vi "Comman1_Main(RemoteLoader).vi"() -> ()   [LabVIEW 2020]
uses:
  RemoteControl_class/RemoteControl.lvclass
  Light_class/Light.lvclass
  GarageDoor_class/GarageDoor.lvclass
  CeilingFan_class/CeilingFan.lvclass
  LightOnCommand_class/LightOnCommand.lvclass
  C:/Projects/OpenGDS_DesignPatterns/Command1/Command_class/Command.lvclass
  LightOffCommand_class/LightOffCommand.lvclass
  GarageDoorOpenCommand_class/GarageDoorOpenCommand.lvclass
  GarageDoorCloseCommand_class/GarageDoorCloseCommand.lvclass
  CeilingFanHighCommand_class/CeilingFanHighCommand.lvclass
  CeilingFanLowCommand_class/CeilingFanLowCommand.lvclass
  Command_class/Command.lvclass
panel:
  in  "stop":bool
  out "error out":errorcluster
  in  "error in (no error)":errorcluster
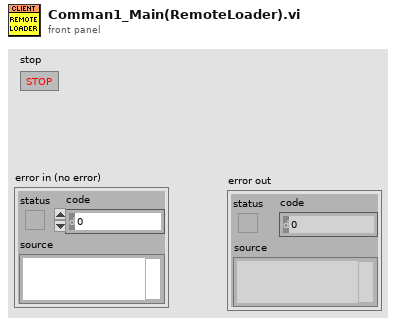
[diagram p1: front panel]
types:
  T1 = cluster{"Remote":refnum<class "RemoteControl.lvclass">, "Light":refnum<class "Light.lvclass">, "GarageDoor":refnum<class "GarageDoor.lvclass">, "CeilingFan":refnum<class "CeilingFan.lvclass">}
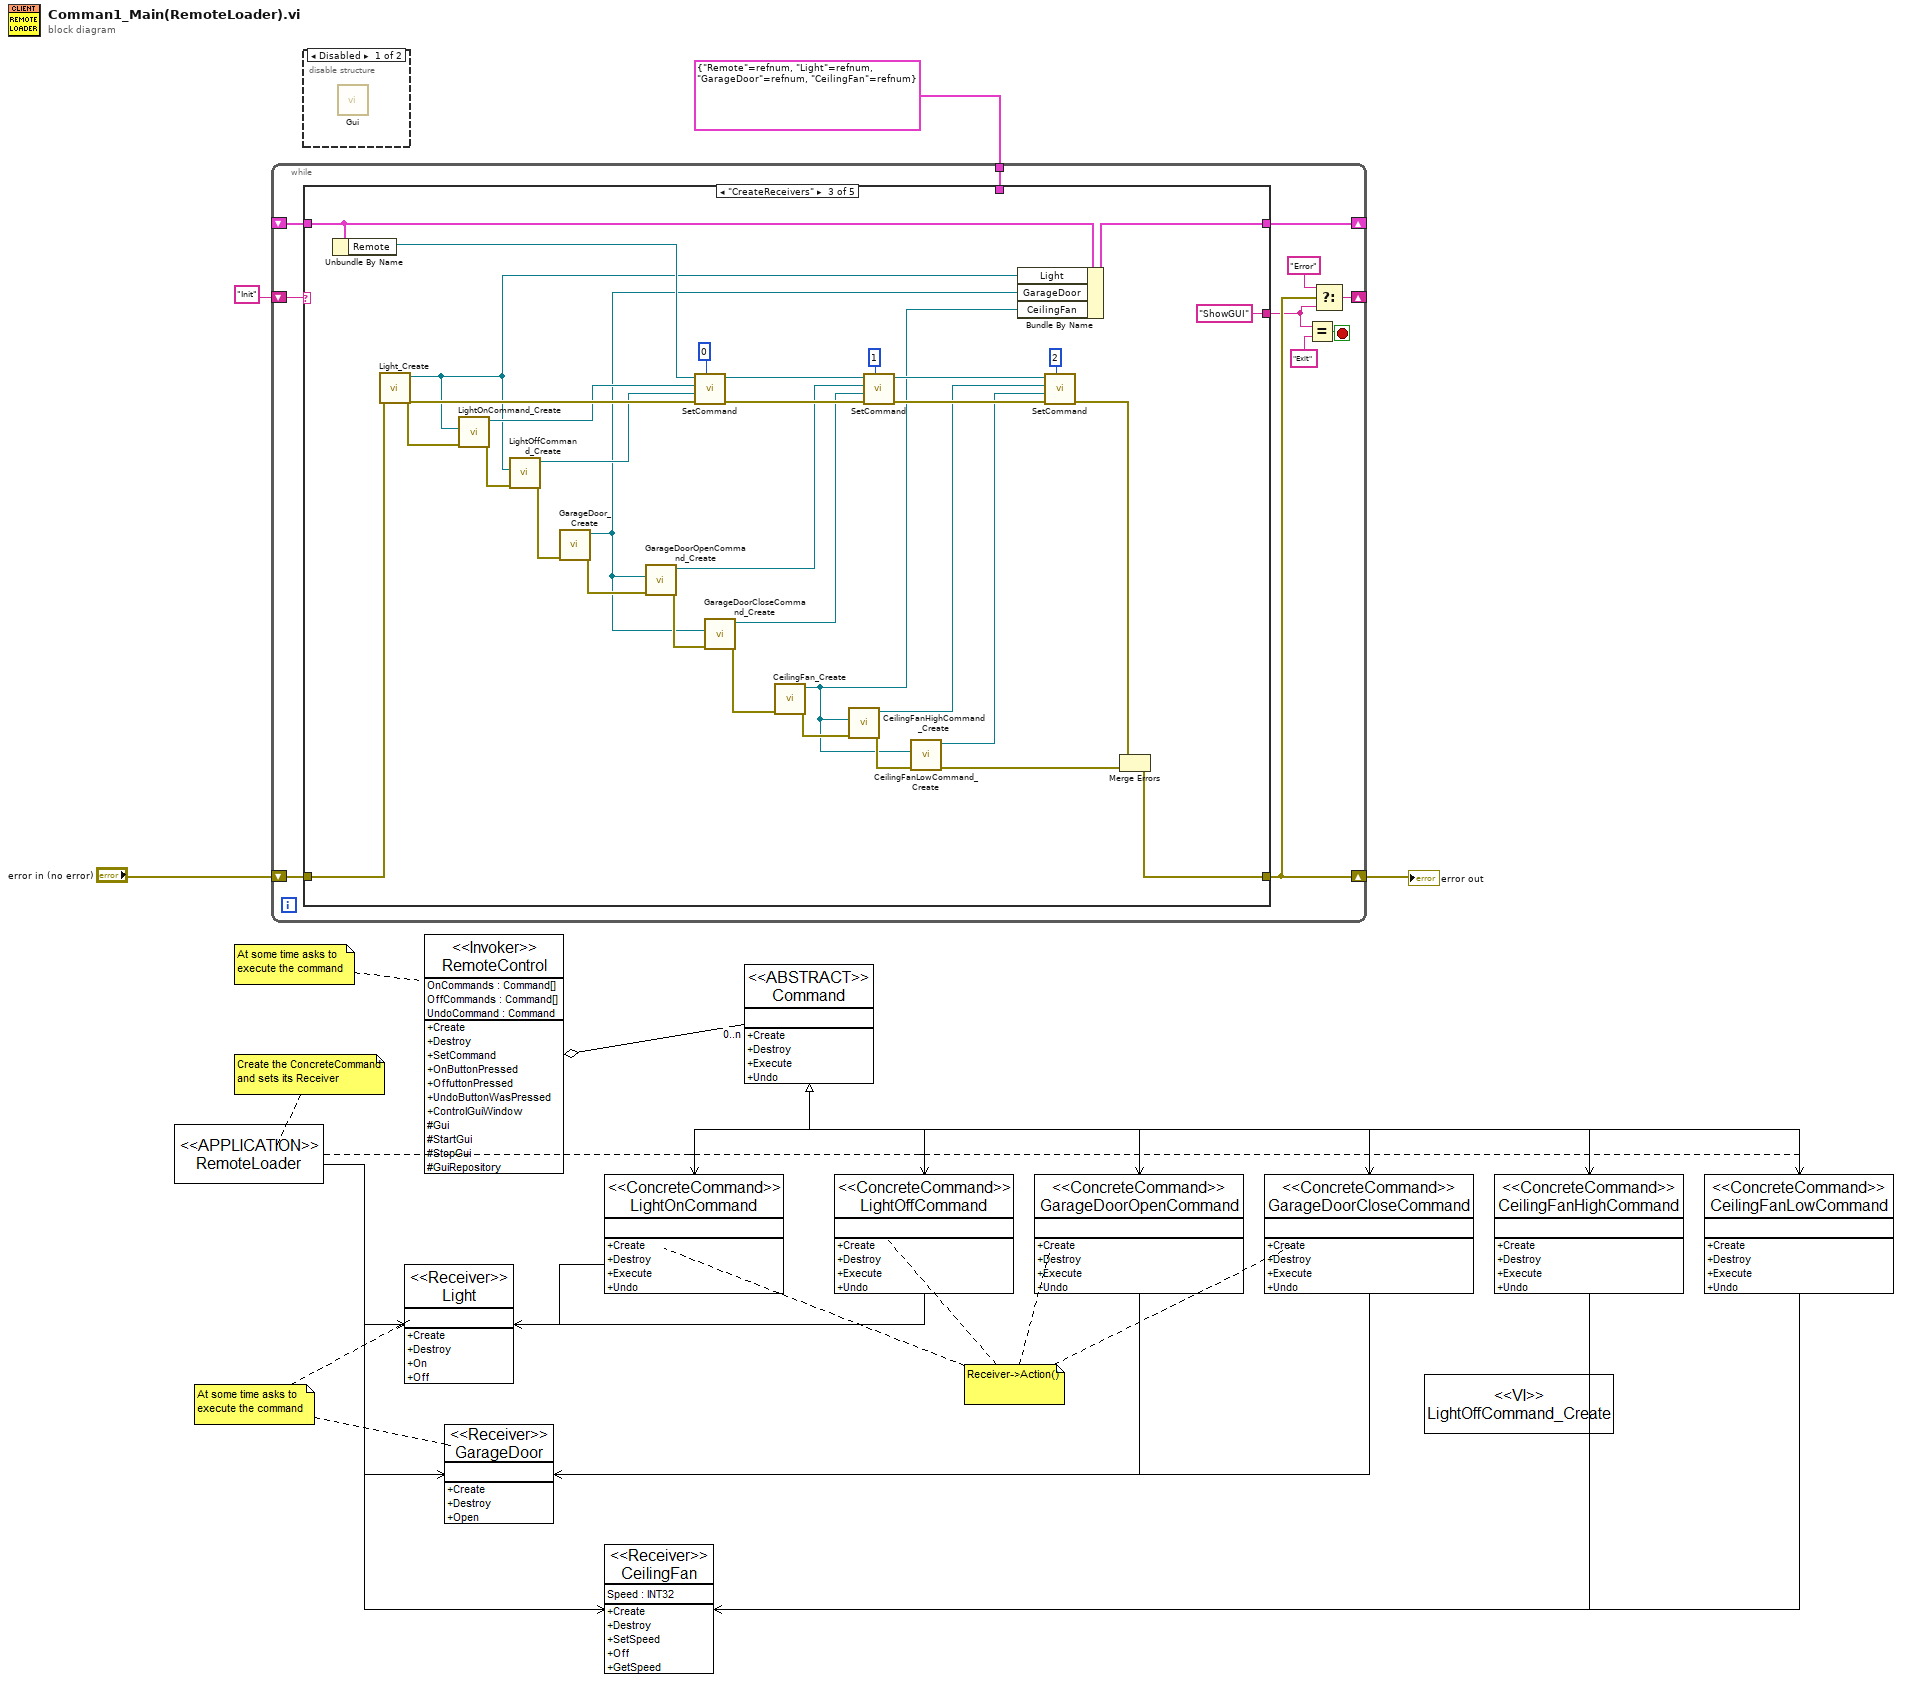
[diagram p0: block diagram]
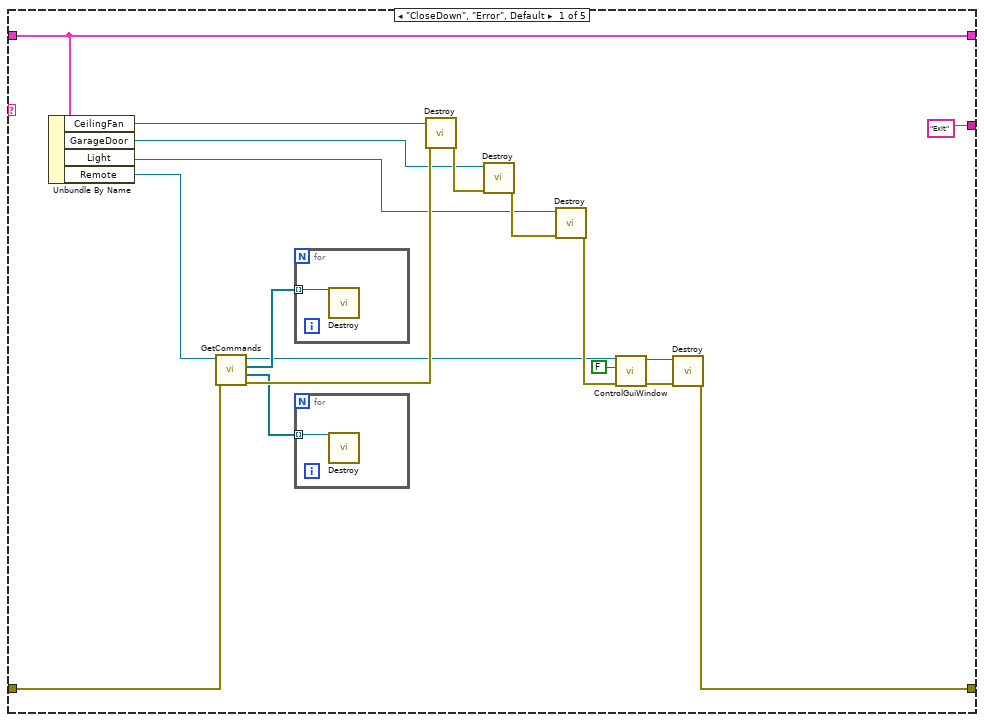
[diagram p3: hidden frame]
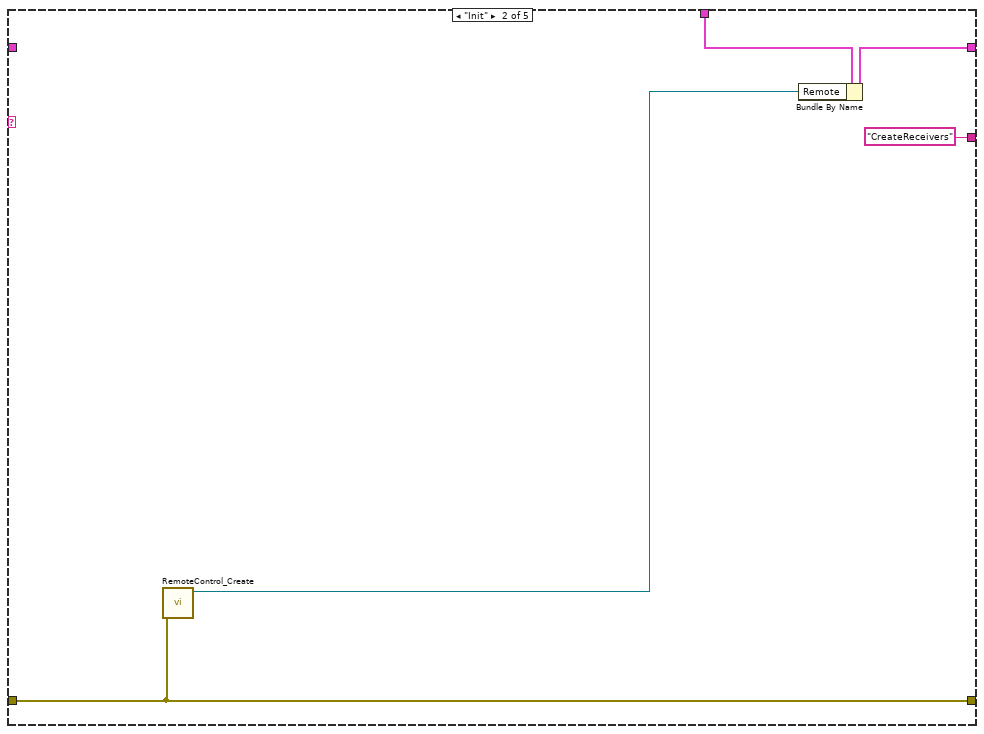
[diagram p4: hidden frame]
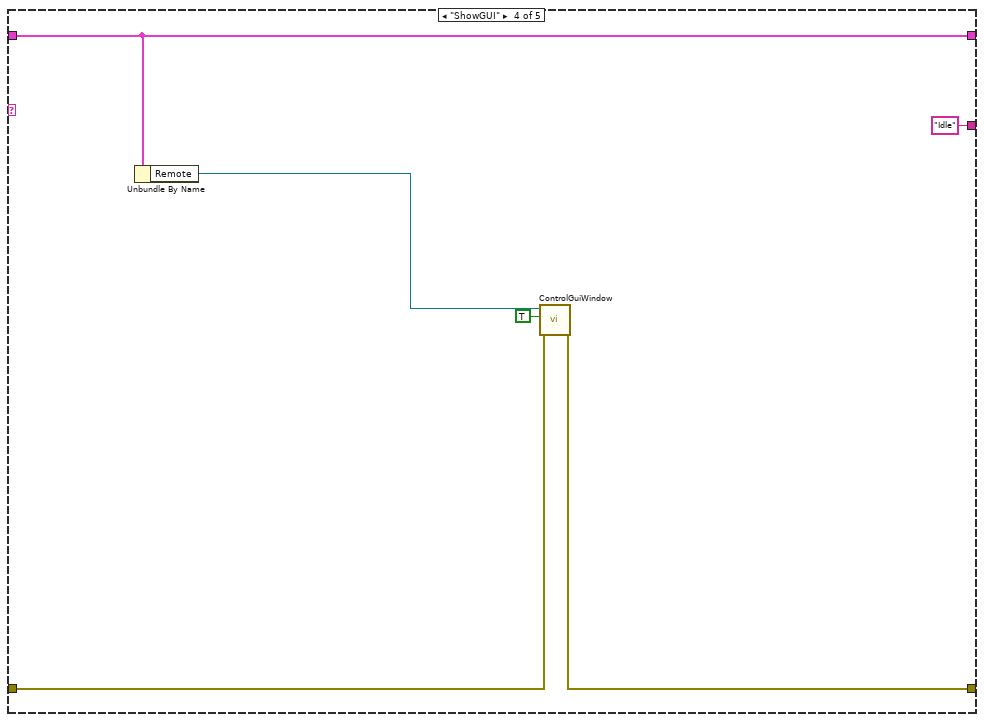
[diagram p5: hidden frame]
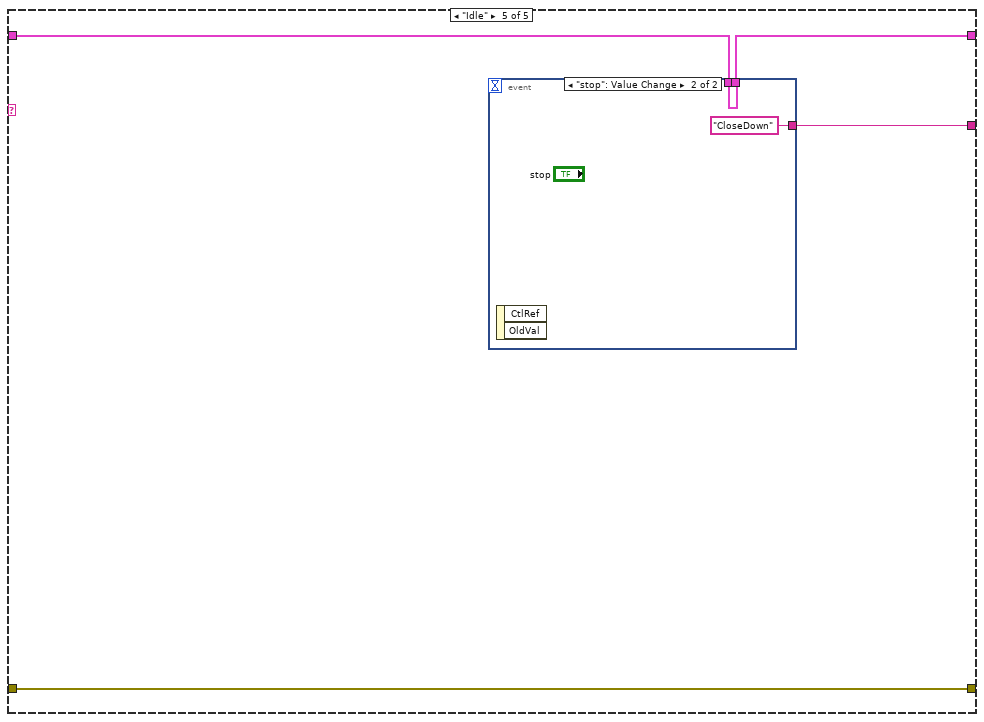
[diagram p6: hidden frame]
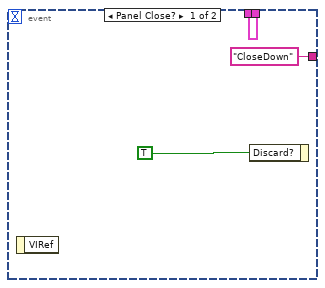
[diagram p7: hidden frame]
diagram:
  n1 = while {
    shift-right: [w14] -> w4
    shift-left: "error in (no error)" -> [w15]
    shift-right: [w12] -> _
    shift-left: "Init" -> [w13]
    shift-right: [w7] -> _
    shift-left: _ -> [w6]
    tunnel: T1 {"Remote"=refnum, "Light"=refnum, "GarageDoor"=refnum, "CeilingFan"=refnum} -> [w5]
    stop <- w11 stop-if-true
    n2 = case shown="\"CreateReceivers\"" w13 {
      tunnel: w15 -> [w28 w40 w68 w78 w82]
      tunnel: [w27 w40 w62 w77 w82] -> w14
      tunnel: ["Exit" "CreateReceivers" "ShowGUI" "Idle" w79] -> w8
      tunnel: [w25 w38 w43 w73 w80] -> w7
      tunnel: w6 -> [w25 _ w44 w73 w81]
      tunnel: w5 -> [_ w36 _ _ _]
      frame "CloseDown", "Error", Default {
        n3 = Unbundle By Name(w25) -> ("CeilingFan"=w24:refnum<class "CeilingFan.lvclass">, "GarageDoor"=w23:refnum<class "GarageDoor.lvclass">, "Light"=w22:refnum<class "Light.lvclass">, "Remote"=w16:refnum<class "RemoteControl.lvclass">)
        n4 = call-dynamic "GetCommands.vi"("error in (no error)"=w28, "reference in"=w16) -> ("error out"=w29:errorcluster, "OfCommands"=w19:refnum<class "Command.lvclass">[], "OnCommands"=w20:refnum<class "Command.lvclass">[], "reference out"=w18:refnum<class "RemoteControl.lvclass">)  [unwired: 6 in]
        n5 = for {
          tunnel: w20 -> [w35] mode=indexing
          n6 = call-dynamic "Destroy.vi"("reference in"=w35) -> ()  [unwired: 9 in, 2 out]
        }
        n7 = for {
          tunnel: w19 -> [w34] mode=indexing
          n8 = call-dynamic "Destroy.vi"("reference in"=w34) -> ()  [unwired: 9 in, 2 out]
        }
        n9 = call-dynamic "Destroy.vi"("error in (no error)"=w29, "reference in"=w24) -> ("error out"=w33:errorcluster)  [unwired: 8 in, 1 out]
        n10 = call-dynamic "Destroy.vi"("error in (no error)"=w33, "reference in"=w23) -> ("error out"=w32:errorcluster)  [unwired: 8 in, 1 out]
        n11 = call-dynamic "Destroy.vi"("error in (no error)"=w32, "reference in"=w22) -> ("error out"=w30:errorcluster)  [unwired: 8 in, 1 out]
        n12 = call "ControlGuiWindow.vi"("error in (no error)"=w30, "ShowProcessWindow"=FALSE, "reference in"=w18) -> ("error out"=w31:errorcluster, "reference out"=w21:refnum<class "RemoteControl.lvclass">)  [unwired: 7 in]
        n13 = call-dynamic "Destroy.vi"("error in (no error)"=w31, "reference in"=w21) -> ("error out"=w27:errorcluster)  [unwired: 8 in, 1 out]
      }
      frame "Init" {
        n14 = call "RemoteControl_Create.vi"("error in (no error)"=w40) -> ("reference out"=w37:refnum<class "RemoteControl.lvclass">)  [unwired: 9 in, 1 out]
        n15 = Bundle By Name(cluster=w36, "Remote"=w37) -> (w38:T1)
      }
      frame "CreateReceivers" {
        n16 = Unbundle By Name(w44) -> ("Remote"=w52:refnum<class "RemoteControl.lvclass">)
        n17 = call "Light_Create.vi"("error in (no error)"=w68) -> ("error out"=w65:errorcluster, "reference out"=w49:refnum<class "Light.lvclass">)  [unwired: 9 in]
        n18 = call "LightOnCommand_Create.vi"("error in (no error)"=w65, "Light"=w49) -> ("error out"=w72:errorcluster, "reference out"=w56:refnum<class "LightOnCommand.lvclass">)  [unwired: 8 in]
        n19 = call "LightOffCommand_Create.vi"("error in (no error)"=w72, "Light"=w49) -> ("error out"=w71:errorcluster, "reference out"=w55:refnum<class "LightOffCommand.lvclass">)  [unwired: 8 in]
        n20 = call "GarageDoor_Create.vi"("error in (no error)"=w71) -> ("error out"=w61:errorcluster, "reference out"=w48:refnum<class "GarageDoor.lvclass">)  [unwired: 9 in]
        n21 = call "GarageDoorOpenCommand_Create.vi"("error in"=w61, "GarageDoor"=w48) -> ("error out"=w60:errorcluster, "reference out"=w42:refnum<class "GarageDoorOpenCommand.lvclass">)  [unwired: 8 in]
        n22 = call-dynamic "SetCommand.vi"("ButtonIndex(0..n)"=0, "error in"=w65, "OffCommand"=w55, "OnCommand"=w56, "reference in"=w52) -> ("error out"=w70:errorcluster, "reference out"=w51:refnum<class "RemoteControl.lvclass">)  [unwired: 5 in]
        n23 = call "GarageDoorCloseCommand_Create.vi"("error in (no error)"=w60, "GarageDoor"=w48) -> ("error out"=w59:errorcluster, "reference out"=w41:refnum<class "GarageDoorCloseCommand.lvclass">)  [unwired: 8 in]
        n24 = call "CeilingFan_Create.vi"("error in (no error)"=w59) -> ("error out"=w67:errorcluster, "reference out"=w47:refnum<class "CeilingFan.lvclass">)  [unwired: 9 in]
        n25 = call "CeilingFanHighCommand_Create.vi"("error in (no error)"=w67, "CeilingFan"=w47) -> ("error out"=w66:errorcluster, "reference out"=w46:refnum<class "CeilingFanHighCommand.lvclass">)  [unwired: 8 in]
        n26 = call-dynamic "SetCommand.vi"("ButtonIndex(0..n)"=1, "error in"=w70, "OffCommand"=w41, "OnCommand"=w42, "reference in"=w51) -> ("error out"=w69:errorcluster, "reference out"=w50:refnum<class "RemoteControl.lvclass">)  [unwired: 5 in]
        n27 = call "CeilingFanLowCommand_Create.vi"("error in (no error)"=w66, "CeilingFan"=w47) -> ("error out"=w64:errorcluster, "reference out"=w45:refnum<class "CeilingFanLowCommand.lvclass">)  [unwired: 8 in]
        n28 = Bundle By Name(cluster=w44, "Light"=w49, "GarageDoor"=w48, "CeilingFan"=w47) -> (w43:T1)
        n29 = call-dynamic "SetCommand.vi"("ButtonIndex(0..n)"=2, "error in"=w69, "OffCommand"=w45, "OnCommand"=w46, "reference in"=w50) -> ("error out"=w63:errorcluster)  [unwired: 5 in, 1 out]
        n30 = Merge Errors(w63, w64) -> (w62:errorcluster)
      }
      frame "ShowGUI" {
        n31 = Unbundle By Name(w73) -> ("Remote"=w76:refnum<class "RemoteControl.lvclass">)
        n32 = call "ControlGuiWindow.vi"("error in (no error)"=w78, "ShowProcessWindow"=TRUE, "reference in"=w76) -> ("error out"=w77:errorcluster)  [unwired: 7 in, 1 out]
      }
      frame "Idle" {
        n33 = event shown="[1] \"stop\": Value Change" {
          selector: _ -> [_ _]
          dyn-events: _ -> [_ _]
          timeout: _ -> [_ _]
          tunnel: w81 -> [w83 w86]
          tunnel: [w83 w86] -> w80
          tunnel: ["CloseDown" "CloseDown"] -> w79
          event Panel Close? {
            n34 = event-data() -> ()  [unwired: 1 in, 1 out]
            n35 = event-data("Discard?"=TRUE) -> ()  [unwired: 1 in, 1 out]
          }
          event "stop": Value Change {
            n36 = event-data() -> ()  [unwired: 1 in, 2 out]
          }
        }
      }
    }
    n37 = Equal?(x=w8, y="Exit") -> (x = y?=w11:bool)
    n38 = Select(t="Error", s=w14, f=w8) -> (s? t:f=w12:string)
  }
  "error out" <- w4
  n39 = disable-structure shown="Disabled" {
    frame Disabled {
      n40 = call "Gui.vi"() -> ()  [unwired: 18 in, 2 out]
    }
    frame Enabled {
    }
  }
